vi "Draw Range Path.vi"(5 "Marker Options":T3={"Color"=24815, "pen"={"Width"=2, "Style"=enum."DashDot"}, "font"={"Font Name"="Arial", "Size"=16, "Strikeout?"=FALSE, "Italic?"=FALSE, "Underline?"=FALSE, "Outline?"=FALSE, "Shadow?"=FALSE, "Bold?"=FALSE, "FontColor"=0}, "caption"=""}, 8 "error in (no error)":errorcluster, 10 "Range Arrows":T1, 11 "GarphView in":refnum<class "GarphView.lvclass">) -> (0 "error out":errorcluster, 3 "GarphView out":refnum<class "GarphView.lvclass">)   [LabVIEW 2020, in "GarphView.lvlib" / "GarphView.lvclass"]
uses:
  GarphView.lvclass
  Range Arrows.ctl
  <vilib>/Utility/miscctls.llb/LVPoint32TypeDef.ctl
  GarphView.lvclass/GarphView.ctl
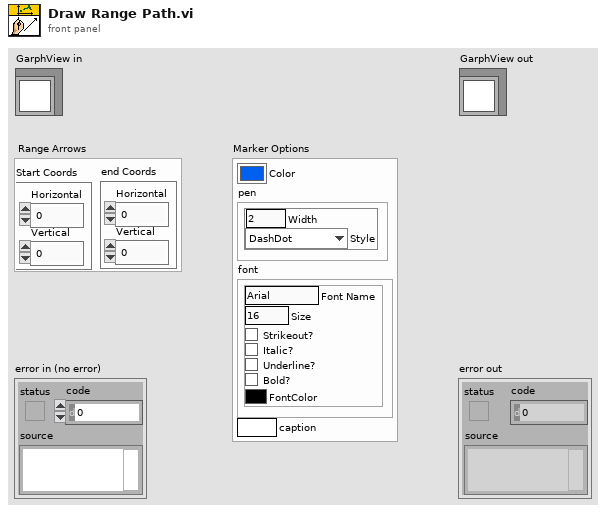
[diagram p1: front panel]
types:
  T1 = typedef "GarphView.lvlib/GarphView.lvclass/Range Arrows.ctl" = cluster{"end Coords":T2, "Start Coords":T2}
  T2 = typedef "LVPoint32TypeDef.ctl" = cluster{"Horizontal":i32, "Vertical":i32}
  T3 = cluster{"Color":u32, "pen":cluster{"Width":u16, "Style":enum32{"Solid", "Dash", "Dot", "DashDot", "DashDotDot"}}, "font":cluster{"Font Name":string, "Size":i16, "Strikeout?":bool, "Italic?":bool, "Underline?":bool, "Outline?":bool, "Shadow?":bool, "Bold?":bool, "FontColor":u32}, "caption":string}
  T4 = typedef "LVRectTypeDef.ctl" = cluster{"Left":i16, "Top":i16, "Right":i16, "Bottom":i16}
  T5 = cluster{"Width":u16, "Style":enum32{"Solid", "Dash", "Dot", "DashDot", "DashDotDot"}}
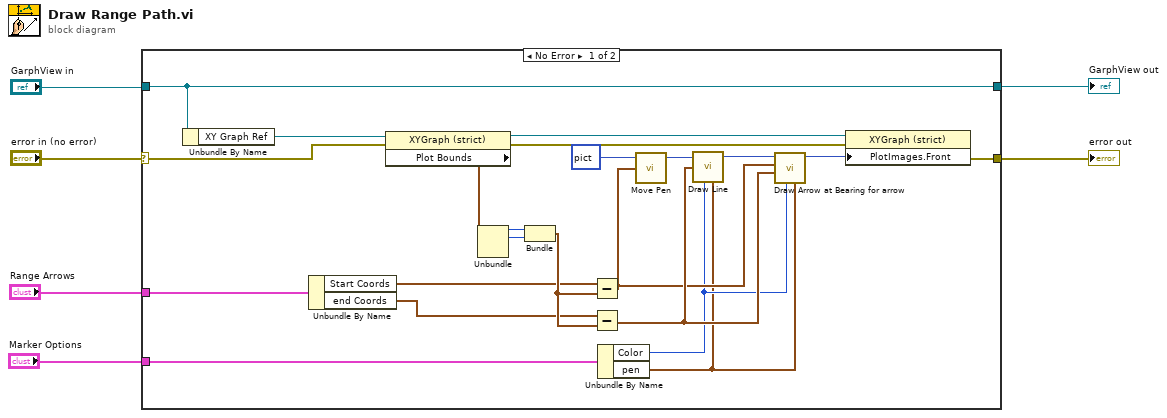
[diagram p0: block diagram]
diagram:
  n1 = case shown="No Error" "error in (no error)" {
    selector: "error in (no error)" -> [w8 w30]
    tunnel: "Marker Options" -> [w23 _]
    tunnel: "GarphView in" -> [w14 w29]
    tunnel: [w15 w30] -> w4
    tunnel: [w14 w29] -> w2
    tunnel: "Range Arrows" -> [w10 _]
    frame No Error {
      n2 = Unbundle By Name(w14) -> ("XY Graph Ref"=w18:refnum<vi>)
      n3 = Unbundle By Name(w10) -> ("Start Coords"=w12:T2, "end Coords"=w11:T2)
      n4 = property class="XYGraph (strict)"(reference=w18, error in=w8) -> (reference out=w17:refnum<vi>, error out=w7:errorcluster, "Plot Bounds"=w13:T4)
      n5 = Unbundle(w13) -> ("Left"=w28:i16, "Top"=w27:i16)  [unwired: 2 out]
      n6 = Bundle("Left"=w28, "Top"=w27) -> (w24:cluster{"Left":i16, "Top":i16})  [unwired: 1 in]
      n7 = Subtract(x=w12, y=w24) -> (x-y=w25:T2)
      n8 = Subtract(x=w11, y=w24) -> (x-y=w26:T2)
      n9 = Unbundle By Name(w23) -> ("Color"=w22:u32, "pen"=w21:T5)
      n10 = call <vilib>:"Move Pen.vi"("new position"=w25, "picture"=picture data[5B]) -> ("new picture"=w20:picture)  [unwired: 3 in]
      n11 = call <vilib>:"Draw Line.vi"("picture"=w20, "end point"=w26, "color(black)"=w22, "pen"=w21) -> ("new picture"=w19:picture)  [unwired: 5 in]
      n12 = call "Draw Arrow at Bearing for arrow.vi"("pen"=w21, "color(black)"=w22, "P2"=w26, "P1"=w25, "new picture in"=w19) -> ("new picture out"=w16:picture)  [unwired: 6 in]
      n13 = property class="XYGraph (strict)"(reference=w17, error in=w7, "PlotImages.Front"=w16) -> (error out=w15:errorcluster)  [unwired: 1 out]
    }
    frame Error {
    }
  }
  "error out" <- w4
  "GarphView out" <- w2
